vi "Send Set Current Record from Keypad.vi"(7 "Message Priority (Normal)":T2=enum."Normal", 8 "error in (no error)":errorcluster, 10 "Keypad":T1, 11 "Message Enqueuer":refnum<class "Message Enqueuer.lvclass">) -> (0 "error out":errorcluster, 3 "Message Enqueuer out":refnum<class "Message Enqueuer.lvclass">)   [LabVIEW 2019, in "ATM Controller.lvlib" / "Set Current Record from Keypad Msg.lvclass"]
doc: "This VI sends the message to an actor."
uses:
  Set Current Record from Keypad Msg.lvclass
  <vilib>/ActorFramework/Message Enqueuer/Message Enqueuer.lvclass
  <vilib>/ActorFramework/Message Enqueuer/Message Priority.ctl
  Simulated User Console Actor/Simulated User Console Actor/Keypad - Cluster.ctl
  C:/Program Files (x86)/National Instruments/LabVIEW 2019/vi.lib/ActorFramework/Message/Message.lvclass
  Set Current Record from Keypad Msg.lvclass/Set Current Record from Keypad Msg.ctl
  <vilib>/ActorFramework/Message Enqueuer/Message Enqueuer.lvclass/Message Enqueuer.ctl
  <vilib>/ActorFramework/Message Priority Queue/Priority Enqueue.vi
  Simulated User Console Actor/Simulated User Console Actor/Simulated User Console Actor.lvclass
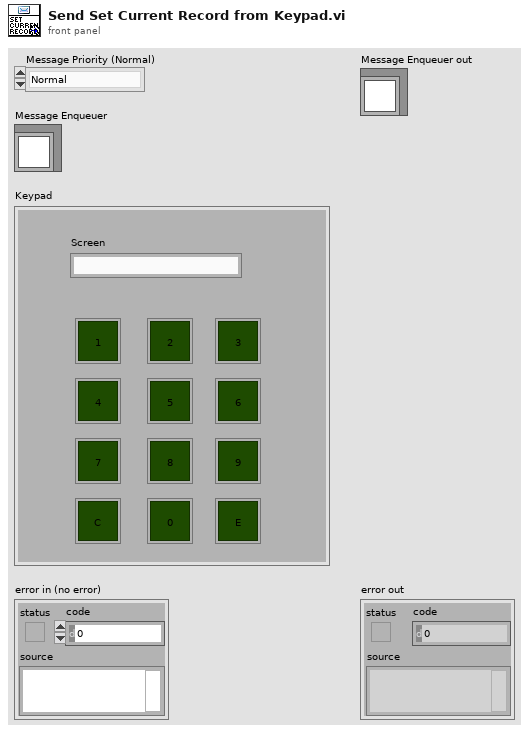
[diagram p1: front panel]
types:
  T1 = typedef "Simulated User Console Actor.lvlib/Simulated User Console Actor.lvclass/Keypad - Cluster.ctl" = cluster{"1":bool, "1 2":bool, "1 3":bool, "1 4":bool, "1 5":bool, "1 6":bool, "1 7":bool, "1 8":bool, "1 9":bool, "C":bool, "1 11":bool, "E":bool, "Screen":string}
  T2 = typedef "Actor Framework.lvlib/Message Enqueuer.lvclass/Message Priority.ctl" = enum16{"Low", "Normal", "High"}
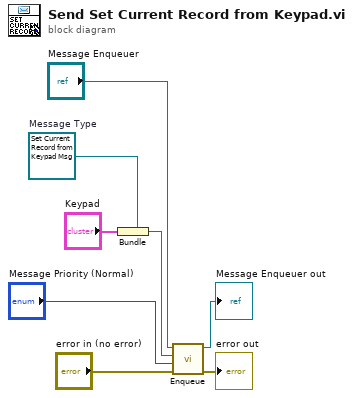
[diagram p0: block diagram]
diagram:
  w5 = refnum<class "Set Current Record from Keypad Msg.lvclass"> refnum  # Message Type
  n1 = Bundle(cluster=w5, "Keypad") -> (w4:refnum<class "Set Current Record from Keypad Msg.lvclass">)
  n2 = call <vilib>:"Enqueue.vi"("error in (no error)"="error in (no error)", "Message Priority (Normal)"="Message Priority (Normal)", "Message"=w4, "Message Enqueuer in"="Message Enqueuer") -> ("error out"=→"error out":errorcluster, "Message Enqueuer out"=→"Message Enqueuer out":refnum<class "Message Enqueuer.lvclass">)  [unwired: 6 in]
